vi "Main Loop.vi"(8 "error in (no error)":errorcluster, 10 "Chart Notifier":refnum<notifier>, 11 "Message Queues":T1) -> (0 "error out":errorcluster)   [LabVIEW 2018, in "Pump Module.lvlib" / "Pump Module Engine.lvlib"]
uses:
  Pump Module Engine.lvlib
  All Message Queues.ctl
  support/Message Queue/Message Cluster.ctl
  State Cluster.ctl
  State Enum.ctl
  Pump Module Settings Cluster.ctl
  Ismatec ISM 831C/Controls/Ismatech Settings Cluster.ctl
  Masterflex 7550-30/Controls/Settings Cluster.ctl
  VICI M50 Party Mode/Settings Cluster.ctl
  Measure Instrument/PID 2 Output Enum.ctl
  Tacmina QI/Tacmina QI DAQ Setting.ctl
  KNF Pump/Settings Cluster plus SIMDOS.ctl
  ASIA Pump/Pump Settings.ctl
  FLOM Pump/Settings Cluster.ctl
  SSI PR Class/SSI PR Settings Cluster.ctl
  Pump Module Display.ctl
  <vilib>/Platform/TimedLoop/XDataNode/timing_clust.ctl
  <vilib>/Platform/TimedLoop/XDataNode/nitl_modes.ctl
  <vilib>/Platform/TimedLoop/XDataNode/wakeup.ctl
  Tag VIs/Tag FGV Operation Enum.ctl
  support/Message Queue/Enqueue Message (Single).vi
  <vilib>/Utility/error.llb/Error Cluster From Error Code.vi
  <vilib>/Platform/TimedLoop/XDataNode/XDataNode.xnode
  <vilib>/ErrorRing/Error Ring.xnode
  support/Message Queue/Message Queue.lvlib
  <vilib>/Platform/TimedLoop/XDataNode/XDNodeRunTimeDep.lvlib
  Pump Module.lvlib
  Ismatec ISM 831C/Ismatec ISM 831C.lvlib
  Masterflex 7550-30/Masterflex 7550-30.lvlib
  Shared Variables/Dynamic Shared Variables.lvlib
  Tacmina QI/Tacmina QI.lvlib
  KNF Pump/KNF SIMDOS.lvlib
  ASIA Pump.lvlib
  VICI M50 Party Mode/VICI M50 Party Mode.lvlib
  FLOM Pump/FLOM Pump.lvlib
  SSI PR Class/SSI PR Pump.lvlib
  support/Support Library.lvlib
panel:
  out "Period (s)":dbl format="%_4g"
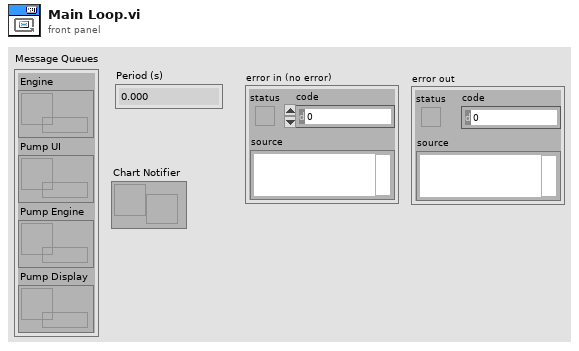
[diagram p1: front panel]
types:
  T1 = typedef "Pump Module.lvlib/All Message Queues.ctl" = cluster{"Engine":refnum<queue>, "Pump UI":refnum<queue>, "Pump Engine":refnum<queue>, "Pump Display":refnum<queue>}
  T2 = typedef "Pump Module.lvlib/Pump Module Display.ctl" = cluster{"Pump On?":enum16{"Off", "On", "Not Initialized"}, "Cycle Period":dbl, "Current Pump Speed":dbl, "Current Pump Pressure":dbl, "Current Pump Flow":dbl, "Output":T3}
  T3 = typedef "PID 2 Output Enum.ctl" = enum16{"Default", "Ismatec ISM 831C", "Masterflex 7550-30", "VICI", "Tacmina QI", "KNF SIMDOS", "ASIA Type C", "FLOM UI-22-11", "SSI PR"}
  T4 = typedef "XDNodeRunTimeDep.lvlib/timing_clust.ctl" = cluster{"Expected End [f-1]":u64, "Actual End [f-1]":u64, "Finished Late? [f-1]":bool, "Expected End [i-1]":u64, "Actual End [i-1]":u64, "Finished Late? [i-1]":bool, "Expected Start [i]":u64, "Actual Start [i]":u64, "Expected Start [f]":u64, "Actual Start [f]":u64, "Source Name":string, "Structure Name":string, "Period":i64, "Deadline":i64, "Offset":i64, "Start":i64, "Priority":i32, "Timeout":i32, "Mode":T5, "Wakeup Reason":T6, "Error":errorcluster, "Source Type":string, "Secondary Source Type":string, "Global End Time":u64, "Global Start Time":u64, "Frame Duration":u64, "Iteration Duration":u64, "Assigned CPU":i32, "I/O Scan Engine Mode":u32}
  T5 = typedef "XDNodeRunTimeDep.lvlib/nitl_modes.ctl" = enum32{"No Change", "Process missed periods, maintain original phase", "Discard missed periods, maintain original phase", "Process missed periods, ignore original phase", "Discard missed periods, ignore original phase"}
  T6 = typedef "XDNodeRunTimeDep.lvlib/wakeup.ctl" = enum32{"Normal", "Aborted", "Asynchronous wakeup", "Timing source error", "Timed loop error", "Timeout"}
  T7 = cluster{"enable? (F)":bool, "name":string, "alarm on":bool, "priority":u32, "ack type":enum16{"Auto", "User", "None", "Each Occurrence"}, "area":string, "description":string, "log? (T)":bool}
  T8 = typedef "Tag FGV Operation Enum.ctl" = enum16{"Init", "Set Notification Queue", "Create Tag", "Commit", "Write Tag (Numeric)", "Write Tag (Boolean)", "Read All Tags", "Read One Tag", "Delete Tag Category", "Set Alarm Parameters (Numeric)", "Set Alarm Parameters (Boolean)", "Enable All Alarms", "Disable All Alarms", "Delete All Tags", "Read Alarms", "Ack Alarm"}
  T9 = enum32{"u32BitField", "bool", "double", "string", "int8", "uint8", "int16", "uint16", "int32", "uint32", "int64", "uint64", "single", "double waveform", "int16 waveform", "array of boolean", "array of int8", "array of uint8", "array of int16", "array of uint16", "array of int32", "array of uint32", "array of int64", "array of uint64", "array of single", "array of double", "array of double waveform", "array of int16 waveform", "array of string", "variant", "timestamp", "fixed point", "custom"}
  T10 = typedef "Pump Module.lvlib/Pump Module Engine.lvlib/State Enum.ctl" = enum16{"Measuring", "Idle", "Paused"}
  T11 = typedef "Pump Module.lvlib/Pump Module Engine.lvlib/State Cluster.ctl" = cluster{"State":T10, "Start Time":timestamp, "Configuration":T12, "Current Time":timestamp, "First Iteration":bool, "Data":cluster{"Pump Speed":dbl, "Pump Pressure":dbl, "Pump Flow":dbl}, "Process Name":string, "Pump On?":enum16{"Off", "On", "Not Initialized"}, "Output Error":bool, "Log Started":bool, "Overpressure Alarming":bool}
  T12 = typedef "Pump Module.lvlib/Pump Module Settings Cluster.ctl" = cluster{"Cycle Period":dbl, "Ismatech":T13, "Masterflex":T14, "Manual Entry":dbl, "VICI Settings":T15, "Output Device":T3, "Tacmina Settings":T16, "KNF SIMDOS Settings":T17, "ASIA Pump C":T18, "FLOM Settings":T19, "Pump Calibration File":path, "Calibration Slope":dbl, "Calibration Y Intercept":dbl, "Pump Cal Enum":u16, "SSI PR Settings":T20}
  T13 = typedef "Ismatec ISM 831C.lvlib/Ismatech Settings Cluster.ctl" = cluster{"VISA resource name":refnum<visa-resource-name>, "Simulated?":bool, "Pump Number":dbl, "Reverse?":bool}
  T14 = typedef "Masterflex 7550-30.lvlib/Settings Cluster.ctl" = cluster{"VISA resource name":refnum<visa-resource-name>, "Simulated?":bool, "Pump Number":dbl, "Reverse?":bool}
  T15 = typedef "VICI M50 Party Mode.lvlib/Settings Cluster.ctl" = cluster{"VISA resource name":refnum<visa-resource-name>, "Simulated?":bool, "Pump Letter":string, "Reverse?":bool}
  T16 = typedef "Tacmina QI.lvlib/Tacmina QI DAQ Setting.ctl" = cluster{"Analog DAQ Task":refnum<k21>, "Digital DAQ Task":refnum<k21>}
  T17 = typedef "KNF SIMDOS.lvlib/Settings Cluster plus SIMDOS.ctl" = cluster{"VISA resource name":refnum<visa-resource-name>, "Simulated?":bool}
  T18 = typedef "ASIA Pump.lvlib/Pump Settings.ctl" = cluster{"ASIA Pump #":i32, "channel":i32, "Simulated":bool}
  T19 = typedef "FLOM Pump.lvlib/Settings Cluster.ctl" = cluster{"VISA resource name":refnum<visa-resource-name>, "Simulated?":bool, "Pump Number":dbl}
  T20 = typedef "SSI PR Pump.lvlib/SSI PR Settings Cluster.ctl" = cluster{"VISA resource name":refnum<visa-resource-name>, "Simulated?":bool}
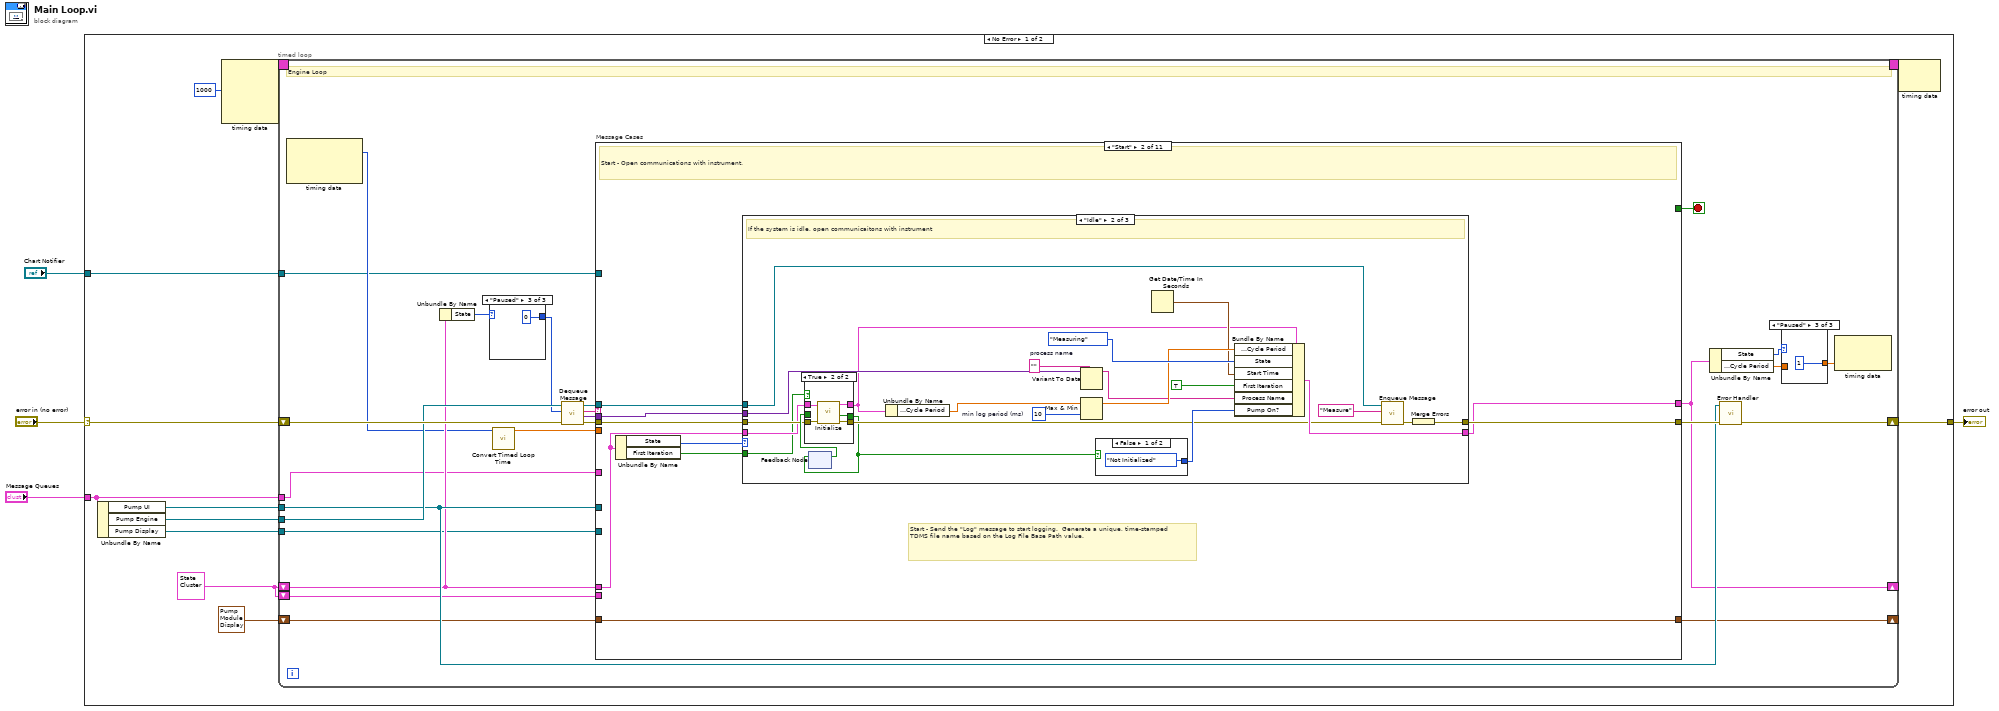
[diagram p0: block diagram]
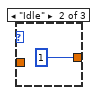
[diagram p3: hidden frame]
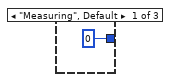
[diagram p4: hidden frame]
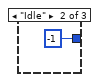
[diagram p5: hidden frame]
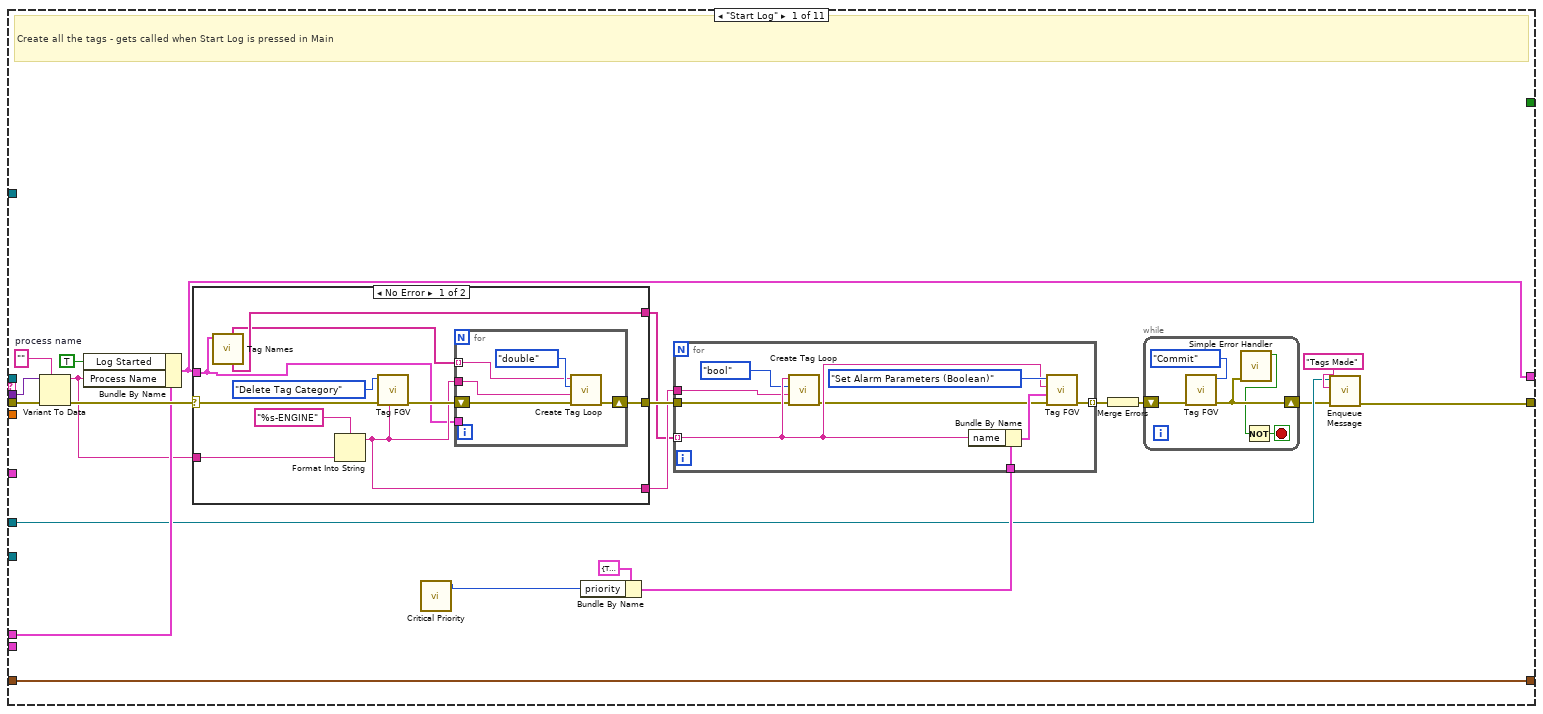
[diagram p6: hidden frame]
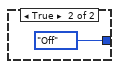
[diagram p10: hidden frame]
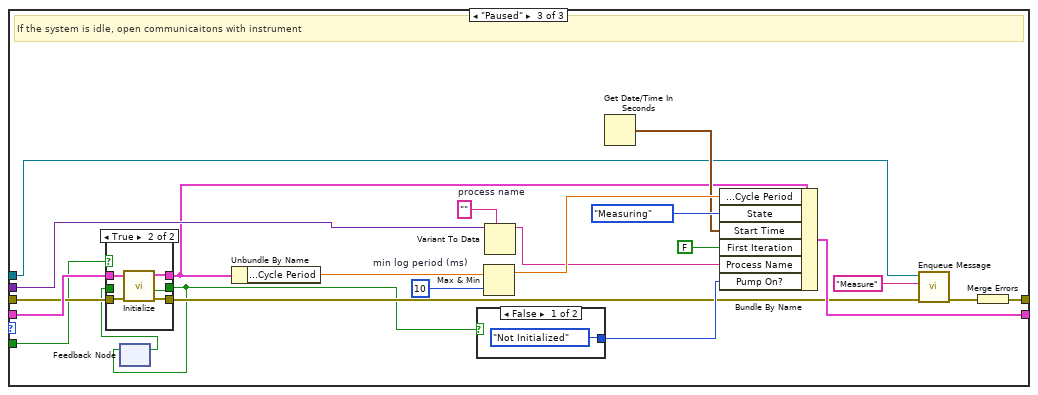
[diagram p11: hidden frame]
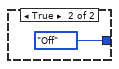
[diagram p13: hidden frame]
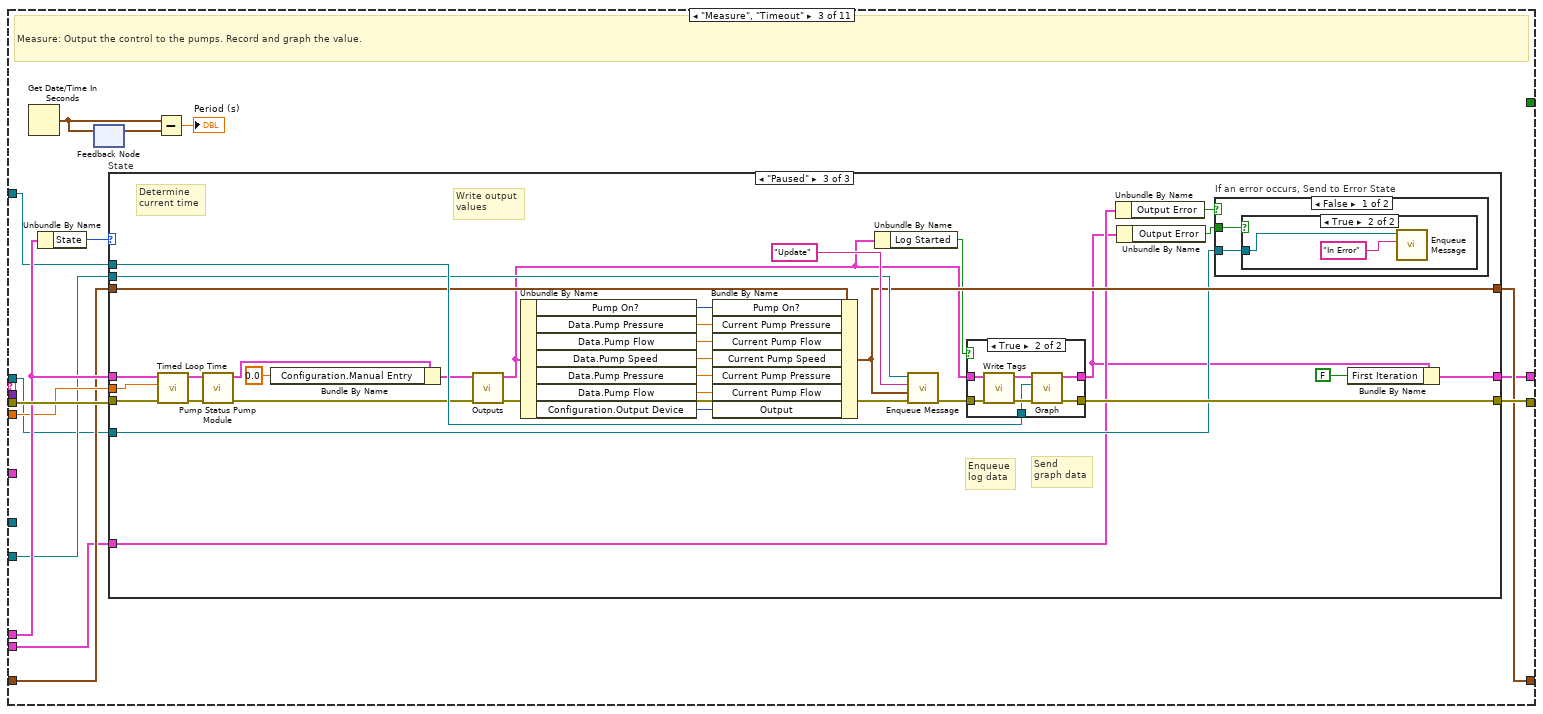
[diagram p14: hidden frame]
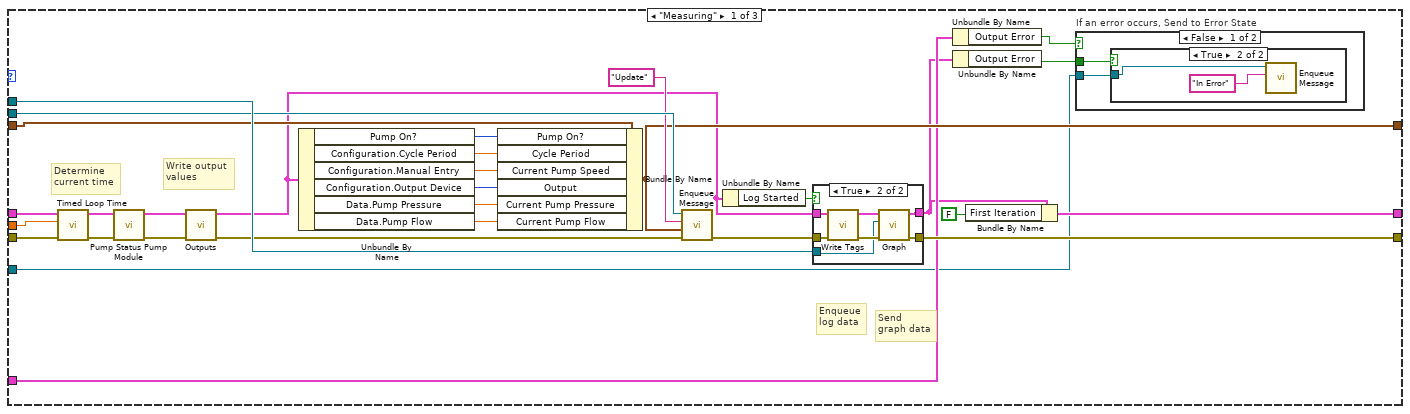
[diagram p15: hidden frame]
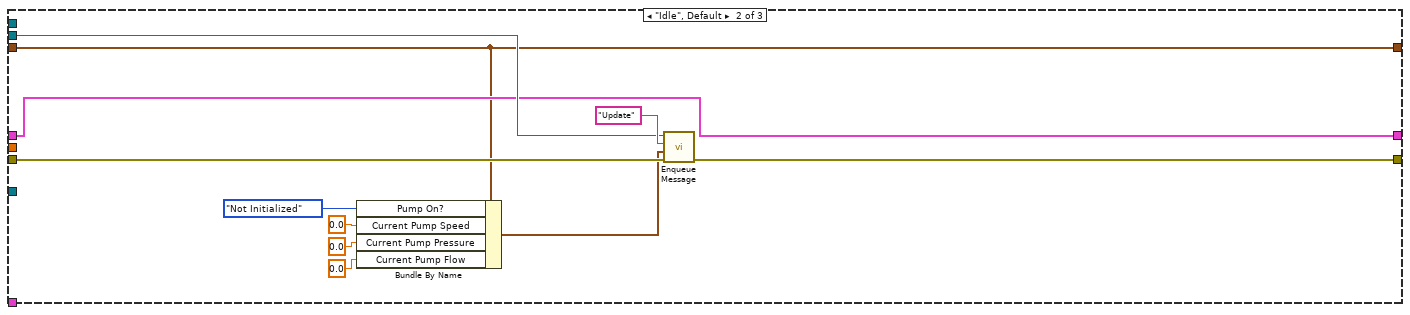
[diagram p19: hidden frame]
diagram:
  n1 = case shown="No Error" "error in (no error)" {
    selector: "error in (no error)" -> [w15 w431]
    tunnel: "Message Queues" -> [w11 _]
    tunnel: [w16 w431] -> w3
    tunnel: "Chart Notifier" -> [w9 _]
    frame No Error {
      w6 = T11 {"State"=enum."Idle", "Start Time"=timestamp(0 s since 1904-01-01), "Configuration"={"Cycle Period"=0.0, "Ismatech"={"VISA resource name"="", "Simulated?"=FALSE, "Pump Number"=1.0, "Reverse?"=FALSE}, "Masterflex"={"VISA resource name"="", "Simulated?"=FALSE, "Pump Number"=1.0, "Reverse?"=FALSE}, "Manual Entry"=0.0, "VICI Settings"={"VISA resource name"="", "Simulated?"=FALSE, "Pump Letter"="", "Reverse?"=FALSE}, "Output Device"=enum."VICI", "Tacmina Settings"={"Analog DAQ Task"="", "Digital DAQ Task"=""}, "KNF SIMDOS Settings"={"VISA resource name"="", "Simulated?"=TRUE}, "ASIA Pump C"={"ASIA Pump #"=0, "channel"=0, "Simulated"=FALSE}, "FLOM Settings"={"VISA resource name"="", "Simulated?"=TRUE, "Pump Number"=0.0}, "Pump Calibration File"=path "", "Calibration Slope"=0.0, "Calibration Y Intercept"=0.0, "Pump Cal Enum"=0, "SSI PR Settings"={"VISA resource name"="", "Simulated?"=FALSE}}, "Current Time"=timestamp(0 s since 1904-01-01), "First Iteration"=FALSE, "Data"={"Pump Speed"=0.0, "Pump Pressure"=0.0, "Pump Flow"=0.0}, "Process Name"="", "Pump On?"=enum."Off", "Output Error"=FALSE, "Log Started"=FALSE, "Overpressure Alarming"=FALSE}
      n2 = Unbundle By Name(w11) -> ("Pump UI"=w14:refnum<queue>, "Pump Engine"=w10:refnum<queue>, "Pump Display"=w8:refnum<queue>)
      n3 = node-c288(i64 1000 ("Period")) -> (w13:T4)  [unwired: 3 in]
      n4 = timed-loop {
        tunnel: w10 -> [w35]
        shift-right: [w17] -> _
        shift-left: w6 -> [w31]
        shift-right: [w33] -> w16
        shift-left: w15 -> [w40]
        tunnel: w14 -> [w32]
        timing: w13 -> [_]
        timing-out: [_] -> w12
        tunnel: w11 -> [w23]
        tunnel: w9 -> [w22]
        tunnel: w8 -> [w21]
        shift-right: [w20] -> _
        shift-left: T2 {"Pump On?"=enum."Off", "Cycle Period"=500.0, "Current Pump Speed"=0.0, "Current Pump Pressure"=0.0, "Current Pump Flow"=0.0, "Output"=enum."Default"} ("PM Display") -> [w19]
        shift-left: w6 -> [w18]
        stop <- w41 stop-if-true
        # "Engine Loop"
        n5 = node-c288() -> (w25:i64)  [unwired: 1 in, 2 out]
        n6 = Unbundle By Name(w31) -> ("State"=w30:T10)
        n7 = case shown="\"Paused\"" w30 {
          tunnel: [0 ("timeout in ms (-1)") -1 ("timeout in ms (-1)") 0 ("timeout in ms (-1)")] -> w29
          frame "Measuring", Default {
          }
          frame "Idle" {
          }
          frame "Paused" {
          }
        }
        n8 = call "Convert Timed Loop Time.vi"("Actual Start [i]"=w25) -> ("ET since start (s)"=w24:dbl)  [unwired: 10 in]
        n9 = call "Dequeue Message.vi"("error in (no error)"=w40, "timeout in ms (-1)"=w29, "Message Queue"=w35) -> ("error out"=w39:errorcluster, "Message Data"=w37:variant, "Message"=w38:string, "dup Message Queue"=w36:refnum<queue>)  [unwired: 5 in]
        n10 = case "Message Cases" shown="\"Start\"" w38 {
          selector: w38 -> [_ _ _ _ _ _ _ _ _ _ w418]
          tunnel: w36 -> [_ w111 w181 _ _ _ w367 _ w379 _ _]
          tunnel: w39 -> [w55 w110 w191 w295 w318 w361 w370 w377 w397 w415 _]
          tunnel: [w59 w112 w192 w299 w322 w357 w372 w376 w392 w414 w419] -> w34
          tunnel: w31 -> [w62 w107 w190 w302 w319 w358 w363 w374 w396 w412 w416]
          tunnel: [w57 w104 w179 w296 w326 w356 w363 w374 w393 w410 w416] -> w17
          tunnel: [_ _ _ _ _ _ TRUE _ _ _ _] -> w41
          tunnel: w37 -> [w72 w108 _ _ _ w362 _ _ _ _ _]
          tunnel: w32 -> [w58 _ _ w304 _ _ w371 _ _ _ _]
          tunnel: w24 -> [_ _ w189 _ _ _ _ _ _ _ _]
          tunnel: w23 -> [_ _ _ _ _ _ _ _ _ _ _]
          tunnel: w22 -> [_ _ w185 _ _ _ _ _ _ _ _]
          tunnel: w21 -> [_ _ w184 w298 w324 _ _ _ w378 _ _]
          tunnel: w19 -> [w73 w106 w183 w297 w321 w359 w364 w375 w387 w413 w417]
          tunnel: [w73 w106 w182 w297 w321 w359 w364 w375 w386 w413 w417] -> w20
          tunnel: w18 -> [_ _ w180 _ _ _ _ _ _ _ _]
          frame "Start Log" {
            w71 = ""  # process name
            # "Create all the tags - gets called when Start Log is pressed in Main"
            n11 = Variant To Data(error in=w55, type=w71, Variant=w72) -> (data=w56:string, error out=w70:errorcluster)
            n12 = Bundle By Name(cluster=w62, "Log Started"=TRUE, "Process Name"=w56) -> (w57:T11)
            n13 = case shown="No Error" w70 {
              selector: w70 -> [w94 w103]
              tunnel: [w97 w103] -> w66
              tunnel: [w92 _] -> w65
              tunnel: [w91 _] -> w64
              tunnel: w57 -> [w88 _]
              tunnel: w56 -> [w90 _]
              frame No Error {
                n14 = call "Tag Names.vi"("State In"=w88) -> ("All Boolean Tags"=w91:string[], "All  Numeric Tags"=w89:string[])  [unwired: 8 in, 1 out]
                n15 = Format Into String(format string="%s-ENGINE", w90) -> (resulting string=w92:string)  [unwired: 2 in, 1 out]
                n16 = call "Tag FGV.vi"("Tag Category"=w92, "error in (no error)"=w94, "Operation"=Tag_FGV_Operation_Enum."Delete Tag Category") -> ("error out"=w93:errorcluster)  [unwired: 3 in, 5 out]
                n17 = for {
                  shift-right: [w98] -> w97
                  shift-left: w93 -> [w99]
                  tunnel: w92 -> [w100]
                  tunnel: w89 -> [w101] mode=indexing
                  tunnel: w88 -> [_]
                  n18 = call "Create Tag Loop.vi"("error in (no error)"=w99, "Tag Category"=w100, "data type"=T9."double", "Tag Name"=w101) -> ("error out"=w98:errorcluster)  [unwired: 7 in]
                }
              }
              frame Error {
              }
            }
            n19 = call "Critical Priority.vi"() -> ("critical priority"=w69:i32)  [unwired: 11 in]
            n20 = Bundle By Name(cluster=T7 {"enable? (F)"=TRUE, "name"="Boolean", "alarm on"=TRUE, "priority"=1, "ack type"=enum."Each Occurrence", "area"="a", "description"="", "log? (T)"=TRUE} ("Boolean alarm settings"), "priority"=w69) -> (w67:T7)
            n21 = for {
              tunnel: w67 -> [w87]
              tunnel: [w86] -> w63 mode=indexing
              tunnel: w64 -> [w83] mode=indexing
              tunnel: w66 -> [w80]
              tunnel: w65 -> [w81]
              n22 = call "Create Tag Loop.vi"("error in (no error)"=w80, "Tag Category"=w81, "data type"=T9."bool", "Tag Name"=w83) -> ("error out"=w79:errorcluster)  [unwired: 7 in]
              n23 = Bundle By Name(cluster=w87, "name"=w83) -> (w85:T7)
              n24 = call "Tag FGV.vi"("error in (no error)"=w79, "Data"=w85, "Tag Name"=w83, "Operation"=Tag_FGV_Operation_Enum."Set Alarm Parameters (Boolean)") -> ("error out"=w86:errorcluster)  [unwired: 2 in, 5 out]
            }
            n25 = Merge Errors(w63) -> (w54:errorcluster)
            n26 = while {
              shift-right: [w76] -> w53
              shift-left: w54 -> [w77]
              stop <- w74 stop-if-true
              n27 = call "Tag FGV.vi"("error in (no error)"=w77, "Operation"=Tag_FGV_Operation_Enum."Commit") -> ("error out"=w76:errorcluster)  [unwired: 4 in, 5 out]
              n28 = call <vilib>:"Simple Error Handler.vi"("error in (no error)"=w76) -> ("error?"=w75:bool)  [unwired: 4 in, 4 out]
              n29 = Not(x=w75) -> (.not. x?=w74:bool)
            }
            n30 = call-poly "Enqueue Message.vi"("error in (no error)"=w53, "Message"="Tags Made", "Message Queue"=w58) -> ("error out"=w59:errorcluster)  [unwired: 7 in, 1 out]
          }
          frame "Start" {
            # "Start - Send the \"Log\" message to start logging.  Generate a unique, time-stamped TDMS file name based on the Log File Base Path value."
            # "Start - Open communications with instrument."
            n31 = Unbundle By Name(w107) -> ("State"=w109:T10, "First Iteration"=w105:bool)
            n32 = case shown="\"Idle\"" w109 {
              tunnel: [w113 w136 w168] -> w112
              tunnel: w111 -> [_ w127 w159]
              tunnel: w110 -> [w113 w120 w151]
              tunnel: w107 -> [w114 w119 w153]
              tunnel: [w114 w134 w166] -> w104
              tunnel: w108 -> [_ w124 w156]
              tunnel: w105 -> [_ w115 w147]
              frame "Measuring", Default {
                # "The system is already running. Ignore the \"Start\" message."
              }
              frame "Idle" {
                w125 = ""  # process name
                w131 = 10  # min log period (ms)
                # "If the system is idle, open communicaitons with instrument"
                n33 = feedback #1() -> (w121:bool)  [unwired: 1 in]
                n34 = case shown="True" w115 {
                  tunnel: w120 -> [w138 w143]
                  tunnel: w119 -> [w139 w144]
                  tunnel: [w139 w142] -> w118
                  tunnel: [w138 w140] -> w117
                  tunnel: [w137 w141] -> w116
                  tunnel: w121 -> [w137 _]
                  frame False {
                  }
                  frame True {
                    n35 = call "Initialize.vi"("error in (no error)"=w143, "State in"=w144) -> ("error out"=w140:errorcluster, "Initialized"=w141:bool, "State out"=w142:T11)  [unwired: 7 in]
                  }
                }
                n36 = feedback-in #1(w116) -> ()
                n37 = Unbundle By Name(w118) -> ("Configuration.Cycle Period"=w130:dbl)
                n38 = Max & Min(x=w130, y=w131) -> (max(x,y)=w129:dbl)  [unwired: 1 out]
                n39 = Variant To Data(type=w125, Variant=w124) -> (data=w123:string)  [unwired: 1 in, 1 out]
                n40 = case shown="False" w116 {
                  tunnel: [enum16{"Off", "On", "Not Initialized"}."Not Initialized" ("Pump On?") enum16{"Off", "On", "Not Initialized"}."Off" ("Pump On?")] -> w122
                  frame False {
                  }
                  frame True {
                  }
                }
                n41 = Get Date/Time In Seconds() -> (seconds since 1Jan1904=w128:timestamp)
                n42 = Bundle By Name(cluster=w118, "Configuration.Cycle Period"=w129, "State"=State_Enum."Measuring", "Start Time"=w128, "First Iteration"=TRUE, "Process Name"=w123, "Pump On?"=w122) -> (w134:T11)
                n43 = call-poly "Enqueue Message.vi"("error in (no error)"=w117, "Message"="Measure", "Message Queue"=w127) -> ("error out"=w132:errorcluster)  [unwired: 7 in, 1 out]
                n44 = Merge Errors(w132) -> (w136:errorcluster)
              }
              frame "Paused" {
                w157 = ""  # process name
                w163 = 10  # min log period (ms)
                # "If the system is idle, open communicaitons with instrument"
                n45 = feedback #2() -> (w148:bool)  [unwired: 1 in]
                n46 = case shown="True" w147 {
                  tunnel: w151 -> [w170 w175]
                  tunnel: w153 -> [w171 w176]
                  tunnel: [w171 w174] -> w152
                  tunnel: [w170 w172] -> w150
                  tunnel: [w169 w173] -> w149
                  tunnel: w148 -> [w169 _]
                  frame False {
                  }
                  frame True {
                    n47 = call "Initialize.vi"("error in (no error)"=w175, "State in"=w176) -> ("error out"=w172:errorcluster, "Initialized"=w173:bool, "State out"=w174:T11)  [unwired: 7 in]
                  }
                }
                n48 = feedback-in #2(w149) -> ()
                n49 = Unbundle By Name(w152) -> ("Configuration.Cycle Period"=w162:dbl)
                n50 = case shown="False" w149 {
                  tunnel: [enum16{"Off", "On", "Not Initialized"}."Not Initialized" ("Pump On?") enum16{"Off", "On", "Not Initialized"}."Off" ("Pump On?")] -> w154
                  frame False {
                  }
                  frame True {
                  }
                }
                n51 = Max & Min(x=w162, y=w163) -> (max(x,y)=w161:dbl)  [unwired: 1 out]
                n52 = Variant To Data(type=w157, Variant=w156) -> (data=w155:string)  [unwired: 1 in, 1 out]
                n53 = Get Date/Time In Seconds() -> (seconds since 1Jan1904=w160:timestamp)
                n54 = Bundle By Name(cluster=w152, "Configuration.Cycle Period"=w161, "State"=State_Enum."Measuring", "Start Time"=w160, "First Iteration"=FALSE, "Process Name"=w155, "Pump On?"=w154) -> (w166:T11)
                n55 = call-poly "Enqueue Message.vi"("error in (no error)"=w150, "Message"="Measure", "Message Queue"=w159) -> ("error out"=w164:errorcluster)  [unwired: 7 in, 1 out]
                n56 = Merge Errors(w164) -> (w168:errorcluster)
              }
            }
          }
          frame "Measure", "Timeout" {
            # "Measure: Output the control to the pumps. Record and graph the value."
            n57 = Get Date/Time In Seconds() -> (seconds since 1Jan1904=w187:timestamp)
            n58 = Unbundle By Name(w190) -> ("State"=w193:T10)
            n59 = feedback-in #3(w187) -> ()
            n60 = feedback #3() -> (w188:timestamp)  [unwired: 1 in]
            n61 = case "State" shown="\"Paused\"" w193 {
              tunnel: w191 -> [w222 w245 w272]
              tunnel: w190 -> [w221 w243 w273]
              tunnel: [w223 w244 w265] -> w192
              tunnel: [w219 w243 w254] -> w179
              tunnel: w189 -> [w220 _ w279]
              tunnel: w185 -> [w217 _ w280]
              tunnel: w184 -> [w214 w246 w276]
              tunnel: w183 -> [w212 w242 w277]
              tunnel: [w209 w242 w264] -> w182
              tunnel: w181 -> [w197 _ w260]
              tunnel: w180 -> [w199 _ w258]
              frame "Measuring" {
                # "Determine\ncurrent time"
                # "Send\ngraph data"
                # "Enqueue\nlog data"
                # "Write output\nvalues"
                n62 = call "Timed Loop Time.vi"("error in (no error)"=w222, "ET since start (s)"=w220, "State in"=w221) -> ("error out"=w208:errorcluster, "State out"=w207:T11)  [unwired: 7 in]
                n63 = call "Pump Status Pump Module.vi"("error in (no error)"=w208, 11:w207) -> ("error out"=w215:errorcluster, "State out"=w216:T11)  [unwired: 8 in]
                n64 = call "Outputs.vi"("error in (no error)"=w215, "State in"=w216) -> ("error out"=w210:errorcluster, "State out"=w203:T11)  [unwired: 8 in]
                n65 = Unbundle By Name(w203) -> ("Pump On?"=w211:enum16{"Off", "On", "Not Initialized"}, "Configuration.Cycle Period"=w205:dbl, "Configuration.Manual Entry"=w204:dbl, "Configuration.Output Device"=w196:T3, "Data.Pump Pressure"=w195:dbl, "Data.Pump Flow"=w194:dbl)
                n66 = Bundle By Name(cluster=w212, "Pump On?"=w211, "Cycle Period"=w205, "Current Pump Speed"=w204, "Output"=w196, "Current Pump Pressure"=w195, "Current Pump Flow"=w194) -> (w209:T2)
                n67 = call-poly "Enqueue Message.vi"("error in (no error)"=w210, "Message Data"=w209, "Message"="Update", "Message Queue"=w214) -> ("error out"=w206:errorcluster)  [unwired: 6 in, 1 out]
                n68 = Unbundle By Name(w203) -> ("Log Started"=w202:bool)
                n69 = case shown="True" w202 {
                  tunnel: [w228 w234] -> w223
                  tunnel: [w229 w233] -> w198
                  tunnel: w217 -> [_ w232]
                  tunnel: w203 -> [w229 w231]
                  tunnel: w206 -> [w228 w230]
                  frame False {
                  }
                  frame True {
                    n70 = call "Write Tags.vi"("error in (no error)"=w230, "State in"=w231) -> ("error out"=w235:errorcluster, "State out"=w236:T11)  [unwired: 8 in]
                    n71 = call "Graph.vi"("error in (no error)"=w235, "notifier out"=w232, "State in"=w236) -> ("error out"=w234:errorcluster, "State out"=w233:T11)  [unwired: 7 in]
                  }
                }
                n72 = Unbundle By Name(w199) -> ("Output Error"=w200:bool)
                n73 = Unbundle By Name(w198) -> ("Output Error"=w201:bool)
                n74 = Bundle By Name(cluster=w198, "First Iteration"=FALSE) -> (w219:T11)
                n75 = case "If an error occurs, Send to Error State" shown="False" w200 {
                  tunnel: w201 -> [w225 _]
                  tunnel: w197 -> [w224 _]
                  frame False {
                    n76 = case shown="True" w225 {
                      tunnel: w224 -> [_ w226]
                      frame False {
                      }
                      frame True {
                        n77 = call-poly "Enqueue Message.vi"("Message"="In Error", "Message Queue"=w226) -> ()  [unwired: 8 in, 2 out]
                      }
                    }
                  }
                  frame True {
                  }
                }
              }
              frame "Idle", Default {
                n78 = Bundle By Name(cluster=w242, "Pump On?"=enum16{"Off", "On", "Not Initialized"}."Not Initialized", "Current Pump Speed"=0.0, "Current Pump Pressure"=0.0, "Current Pump Flow"=0.0) -> (w241:T2)
                n79 = call-poly "Enqueue Message.vi"("error in (no error)"=w245, "Message Data"=w241, "Message"="Update", "Message Queue"=w246) -> ("error out"=w244:errorcluster)  [unwired: 6 in, 1 out]
              }
              frame "Paused" {
                # "Determine\ncurrent time"
                # "Write output\nvalues"
                # "Send\ngraph data"
                # "Enqueue\nlog data"
                n80 = call "Timed Loop Time.vi"("error in (no error)"=w272, "ET since start (s)"=w279, "State in"=w273) -> ("error out"=w269:errorcluster, "State out"=w271:T11)  [unwired: 7 in]
                n81 = call "Pump Status Pump Module.vi"("error in (no error)"=w269, 11:w271) -> ("error out"=w268:errorcluster, "State out"=w270:T11)  [unwired: 8 in]
                n82 = Bundle By Name(cluster=w270, "Configuration.Manual Entry"=0.0) -> (w274:T11)
                n83 = call "Outputs.vi"("error in (no error)"=w268, "State in"=w274) -> ("error out"=w267:errorcluster, "State out"=w253:T11)  [unwired: 8 in]
                n84 = Unbundle By Name(w253) -> ("Pump On?"=w263:enum16{"Off", "On", "Not Initialized"}, "Data.Pump Pressure"=w262:dbl, "Data.Pump Flow"=w261:dbl, "Data.Pump Speed"=w251:dbl, "Data.Pump Pressure"=w250:dbl, "Data.Pump Flow"=w248:dbl, "Configuration.Output Device"=w249:T3)
                n85 = Bundle By Name(cluster=w277, "Pump On?"=w263, "Current Pump Pressure"=w262, "Current Pump Flow"=w261, "Current Pump Speed"=w251, "Current Pump Pressure"=w250, "Current Pump Flow"=w248, "Output"=w249) -> (w264:T2)
                n86 = Unbundle By Name(w253) -> ("Log Started"=w252:bool)
                n87 = call-poly "Enqueue Message.vi"("error in (no error)"=w267, "Message Data"=w264, "Message"="Update", "Message Queue"=w276) -> ("error out"=w266:errorcluster)  [unwired: 6 in, 1 out]
                n88 = case shown="True" w252 {
                  tunnel: w280 -> [_ w287]
                  tunnel: w266 -> [w281 w286]
                  tunnel: [w281 w285] -> w265
                  tunnel: w253 -> [w282 w284]
                  tunnel: [w282 w283] -> w255
                  frame False {
                  }
                  frame True {
                    n89 = call "Write Tags.vi"("error in (no error)"=w286, "State in"=w284) -> ("error out"=w289:errorcluster, "State out"=w288:T11)  [unwired: 8 in]
                    n90 = call "Graph.vi"("error in (no error)"=w289, "notifier out"=w287, "State in"=w288) -> ("error out"=w285:errorcluster, "State out"=w283:T11)  [unwired: 7 in]
                  }
                }
                n91 = Unbundle By Name(w258) -> ("Output Error"=w257:bool)
                n92 = Unbundle By Name(w255) -> ("Output Error"=w259:bool)
                n93 = case "If an error occurs, Send to Error State" shown="False" w257 {
                  tunnel: w259 -> [w291 _]
                  tunnel: w260 -> [w290 _]
                  frame False {
                    n94 = case shown="True" w291 {
                      tunnel: w290 -> [_ w293]
                      frame False {
                      }
                      frame True {
                        n95 = call-poly "Enqueue Message.vi"("Message"="In Error", "Message Queue"=w293) -> ()  [unwired: 8 in, 2 out]
                      }
                    }
                  }
                  frame True {
                  }
                }
                n96 = Bundle By Name(cluster=w255, "First Iteration"=FALSE) -> (w254:T11)
              }
            }
            n97 = Subtract(x=w187, y=w188) -> (x-y=→"Period (s)":dbl)
          }
          frame "Stop" {
            # "Stop - Flush the message queue of any pending \"Log\" messages. Call 'Flush Data to Log File.vi' so any pending data is not lost."
            n98 = call <vilib>:"Clear Errors.vi"("error in (no error)"=w295) -> ("error out"=w294:errorcluster)  [unwired: 5 in, 1 out]
            n99 = Unbundle By Name(w302) -> ("State"=w303:T10)
            n100 = case shown="\"Measuring\", Default" w303 {
              tunnel: [w309 w315] -> w300
              tunnel: w294 -> [w306 w315]
              tunnel: w304 -> [w313 _]
              tunnel: w302 -> [w307 w314]
              tunnel: [w311 w314] -> w296
              frame "Measuring", Default {
                # "If the system is logging, stop logging."
                n101 = call "Close.vi"("error in (no error)"=w306, "State in"=w307) -> ("error out"=w305:errorcluster, "State out"=w308:T11)  [unwired: 8 in]
                n102 = Bundle By Name(cluster=w308, "State"=State_Enum."Idle") -> (w311:T11)
                n103 = call-poly "Enqueue Message.vi"("error in (no error)"=w305, "Message"="Logging Stopped", "Message Queue"=w313) -> ("error out"=w309:errorcluster)  [unwired: 7 in, 1 out]
              }
              frame "Idle" {
                # "The system is already idle. Ignore the \"Stop\" message."
              }
            }
            n104 = call-poly "Enqueue Message.vi"("error in (no error)"=w300, "Message Data"=w297, "Message"="Update", "Message Queue"=w298) -> ("error out"=w299:errorcluster)  [unwired: 6 in, 1 out]
          }
          frame "Pause" {
            # "Stop - Flush the message queue of any pending \"Log\" messages. Call 'Flush Data to Log File.vi' so any pending data is not lost."
            n105 = Unbundle By Name(w319) -> ("State"=w327:T10, "First Iteration"=w320:bool)
            n106 = case shown="True" w320 {
              tunnel: w319 -> [w328 w332]
              tunnel: [w328 w336] -> w317
              tunnel: w318 -> [w329 w333]
              tunnel: [w329 w334] -> w316
              frame False {
              }
              frame True {
                # "If we start on a pause condition, initialize the pump"
                n107 = call "Initialize.vi"("error in (no error)"=w333, "State in"=w332) -> ("error out"=w334:errorcluster, "Initialized"=w335:bool, "State out"=w331:T11)  [unwired: 7 in]
                n108 = case shown="True" w335 {
                  tunnel: [enum16{"Off", "On", "Not Initialized"}."Not Initialized" ("Pump On?") enum16{"Off", "On", "Not Initialized"}."Off" ("Pump On?")] -> w337
                  tunnel: [_ FALSE] -> w330
                  frame False {
                  }
                  frame True {
                  }
                }
                n109 = Bundle By Name(cluster=w331, "Pump On?"=w337, "First Iteration"=w330) -> (w336:T11)
              }
            }
            n110 = case shown="\"Measuring\", Default" w327 {
              tunnel: [w341 w350 w354] -> w323
              tunnel: w316 -> [w345 w350 w354]
              tunnel: w317 -> [w342 w348 w352]
              tunnel: [w343 w347 w351] -> w326
              frame "Measuring", Default {
                # "If the system is logging, stop logging."
                n111 = call "Pause.vi"("error in (no error)"=w345, "State in"=w342) -> ("error out"=w341:errorcluster, "State out"=w344:T11)  [unwired: 8 in]
                n112 = Bundle By Name(cluster=w344, "State"=State_Enum."Paused") -> (w343:T11)
              }
              frame "Idle" {
                # "The system is already idle. Ignore the \"Stop\" message."
                n113 = Bundle By Name(cluster=w348, "State"=State_Enum."Paused") -> (w347:T11)
              }
              frame "Paused" {
                n114 = Bundle By Name(cluster=w352, "State"=State_Enum."Paused") -> (w351:T11)
              }
            }
            n115 = call-poly "Enqueue Message.vi"("error in (no error)"=w323, "Message Data"=w321, "Message"="Update", "Message Queue"=w324) -> ("error out"=w322:errorcluster)  [unwired: 6 in, 1 out]
          }
          frame "Update Settings" {
            w360 = T12 {"Cycle Period"=0.0, "Ismatech"={"VISA resource name"="", "Simulated?"=FALSE, "Pump Number"=1.0, "Reverse?"=FALSE}, "Masterflex"={"VISA resource name"="", "Simulated?"=FALSE, "Pump Number"=1.0, "Reverse?"=FALSE}, "Manual Entry"=0.0, "VICI Settings"={"VISA resource name"="", "Simulated?"=FALSE, "Pump Letter"="", "Reverse?"=FALSE}, "Output Device"=enum."VICI", "Tacmina Settings"={"Analog DAQ Task"="", "Digital DAQ Task"=""}, "KNF SIMDOS Settings"={"VISA resource name"="", "Simulated?"=TRUE}, "ASIA Pump C"={"ASIA Pump #"=0, "channel"=0, "Simulated"=FALSE}, "FLOM Settings"={"VISA resource name"="", "Simulated?"=TRUE, "Pump Number"=0.0}, "Pump Calibration File"=path "", "Calibration Slope"=0.0, "Calibration Y Intercept"=0.0, "Pump Cal Enum"=0, "SSI PR Settings"={"VISA resource name"="", "Simulated?"=FALSE}}  # Configuration
            # "New settings are available, update the current ones stored in the shift register with the settings sent as part of the message"
            n116 = Variant To Data(error in=w361, type=w360, Variant=w362) -> (data=w355:T12, error out=w357:errorcluster)
            n117 = Bundle By Name(cluster=w358, "Configuration"=w355) -> (w356:T11)
          }
          frame "Exit" {
            # "Release the Logging queue reference"
            # "Don't check the error out. The UI message queue may have already been released."
            # "Stop the VI"
            # "Exit - Send the Exit message to the UI Message Handler.  Call 'Flush Data to Log File.vi' so any pending data is not lost."
            n118 = Release Queue(queue=w367, error in (no error)=w370) -> (error out=w366:errorcluster)  [unwired: 1 in, 2 out]
            n119 = call-poly "Enqueue Message.vi"("Priority Message? (F)"=TRUE, "Message"="Exit", "Message Queue"=w371) -> ("error out"=w365:errorcluster)  [unwired: 7 in, 1 out]
            n120 = call <vilib>:"Clear Errors.vi"("error in (no error)"=w365) -> ()  [unwired: 5 in, 2 out]
            n121 = Merge Errors(w366) -> (w372:errorcluster)
          }
          frame "---Copy This Frame---" {
            # "Duplicate this frame when creating new messages.  Change this comment in the duplicated frame to describe this message."
            n122 = Merge Errors(w377) -> (w376:errorcluster)
          }
          frame "In Error" {
            # "If we have a disconnect Error we will go to this state, and attempt to reconnect and get back to the pre-error state"
            n123 = Merge Errors(w397) -> (w394:errorcluster)
            n124 = call "Initialize.vi"("error in (no error)"=w394, "State in"=w396) -> ("error out"=w390:errorcluster, "Initialized"=w395:bool, "State out"=w388:T11)  [unwired: 7 in]
            n125 = Unbundle By Name(w388) -> ("Pump On?"=w380:enum16{"Off", "On", "Not Initialized"}, "Configuration.Cycle Period"=w381:dbl, "Data.Pump Speed"=w382:dbl, "Data.Pump Pressure"=w383:dbl, "Data.Pump Flow"=w384:dbl, "Configuration.Output Device"=w385:T3)
            n126 = Bundle By Name(cluster=w387, "Pump On?"=w380, "Cycle Period"=w381, "Current Pump Speed"=w382, "Current Pump Pressure"=w383, "Current Pump Flow"=w384, "Output"=w385) -> (w386:T2)
            n127 = call-poly "Enqueue Message.vi"("error in (no error)"=w390, "Message Data"=w386, "Message"="Update", "Message Queue"=w378) -> ("error out"=w389:errorcluster)  [unwired: 6 in, 1 out]
            n128 = case shown="False" w395 {
              tunnel: w379 -> [w402 w406]
              tunnel: w389 -> [w401 w405]
              tunnel: [w399 w408] -> w393
              tunnel: w388 -> [w399 w408]
              tunnel: [w398 w404] -> w392
              frame False {
                n129 = Wait (ms)(milliseconds to wait=u32 5000) -> ()  [unwired: 1 out]
                n130 = call-poly "Enqueue Message.vi"("error in (no error)"=w401, "Message"="In Error", "Message Queue"=w402) -> ("error out"=w398:errorcluster)  [unwired: 7 in, 1 out]
              }
              frame True {
                n131 = call-poly "Enqueue Message.vi"("error in (no error)"=w405, "Message"="Measure", "Message Queue"=w406) -> ("error out"=w404:errorcluster)  [unwired: 7 in, 1 out]
              }
            }
          }
          frame "Initialize" {
            # "Duplicate this frame when creating new messages.  Change this comment in the duplicated frame to describe this message."
            n132 = Merge Errors(w415) -> (w414:errorcluster)
            n133 = Bundle By Name(cluster=w412, "Log Started"=FALSE, "First Iteration"=TRUE) -> (w410:T11)
          }
          frame Default {
            # "'Default' case only runs if there is a message that isn't defined in any of the other cases.  Output a programming error."
            n134 = xnode "Error Ring"("parameter 0"=w418) -> ("error out"=w419:errorcluster)
          }
        }
        n135 = Unbundle By Name(w17) -> ("State"=w28:T10, "Configuration.Cycle Period"=w26:dbl)
        n136 = call "Error Handler.vi"("error in (no error)"=w34, "Message Queue"=w32) -> ("dup error in"=w33:errorcluster)  [unwired: 8 in, 1 out]
        n137 = case shown="\"Paused\"" w28 {
          tunnel: [w42 1 1] -> w27
          tunnel: w26 -> [w42 _ _]
          frame "Measuring" {
          }
          frame "Idle" {
          }
          frame "Paused" {
          }
        }
        n138 = node-c288(w27) -> ()  [unwired: 1 in, 1 out]
      }
      n139 = node-c288(w12) -> ()  [unwired: 1 out]
    }
    frame Error {
    }
  }
  "error out" <- w3
